vi "test.vi"() -> ()   [LabVIEW 2010, in "GenericAnalogOut.lvclass"]
uses:
  GenericAnalogOut.lvclass
  common/classes/ErrorController/ErrorController/ErrorController.lvclass
  common/classes/ErrorController/ErrorController/class_data.vi
  common/classes/GenericComponent/GenericComponent/GenericComponent.lvclass
panel:
  out "error loaded?":bool
  in  "create button":bool
  in  "set button":bool
  in  "output voltage":dbl[unit]
  in  "stop button":bool
  # "Test panel for AnalogOut components"
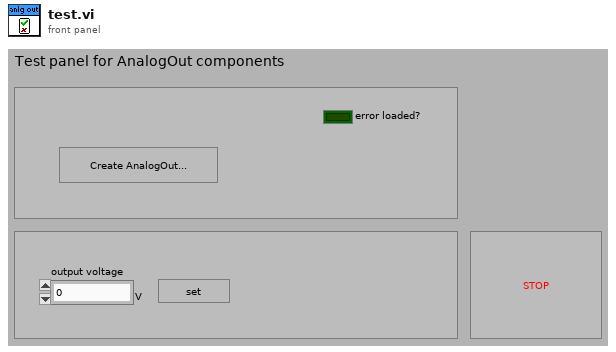
[diagram p1: front panel]
types:
  T1 = typedef "XComponentSpecification.xctl/data.ctl" = cluster{"class path":string, "configuration":string, "label":string, "settings name":string}
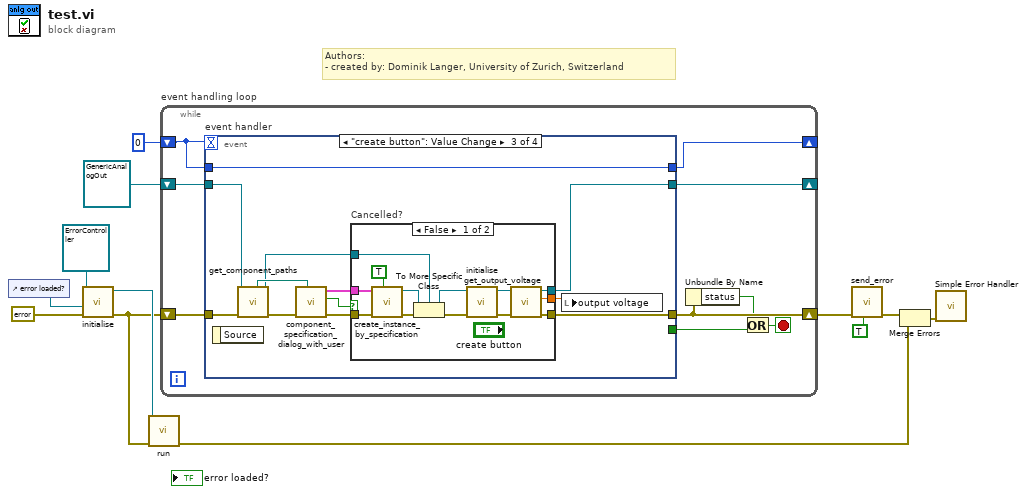
[diagram p0: block diagram]
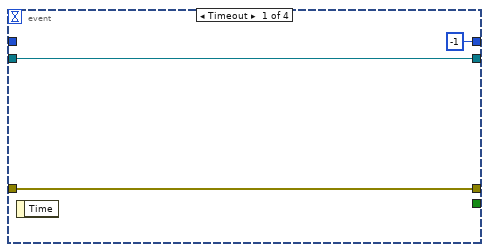
[diagram p2: hidden frame]
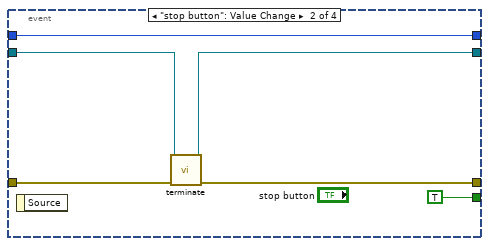
[diagram p3: hidden frame]
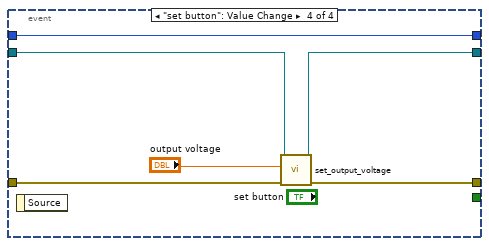
[diagram p5: hidden frame]
diagram:
  # "Authors: \n- created by: Dominik Langer, University of Zurich, Switzerland"
  n1 = control-ref of="error loaded?"() -> (w9:refnum<vi>)
  n2 = call-dynamic "initialise.vi"("error in (no error)"=errorcluster {"status"=FALSE, "code"=0, "source"=""} ("error out"), "error boolean"=w9, "ErrorController in"=refnum<class "ErrorController.lvclass"> refnum ("ErrorController.lvclass")) -> ("error out"=w2:errorcluster, "ErrorController out"=w8:refnum<class "ErrorController.lvclass">)  [unwired: 7 in]
  n3 = call "run.vi"("error in (no error)"=w2, "ErrorController in"=w8) -> ("error out"=w3:errorcluster)  [unwired: 8 in, 1 out]
  n4 = while "event handling loop" {
    shift-right: [w16] -> w7
    shift-left: w2 -> [w21]
    shift-right: [w19] -> _
    shift-left: 0 -> [w20]
    shift-right: [w17] -> _
    shift-left: refnum<class "GenericAnalogOut.lvclass"> refnum ("GenericAnalogOut.lvclass") -> [w18]
    stop <- w13 stop-if-true
    n5 = event "event handler" shown="[2] \"create button\": Value Change" {
      selector: _ -> [_ _ _ _]
      dyn-events: _ -> [_ _ _ _]
      timeout: w20 -> [_ _ _ _]
      tunnel: w21 -> [w23 w26 w36 w62]
      tunnel: [w23 w25 w40 w61] -> w16
      tunnel: [-1 w30 w42 w63] -> w19
      tunnel: w20 -> [_ w30 w42 w63]
      tunnel: w18 -> [w22 w28 w34 w60]
      tunnel: [w22 w27 w39 w59] -> w17
      tunnel: [_ TRUE _ _] -> w14
      event Timeout {
        n6 = event-data() -> ()  [unwired: 2 out]
      }
      event "stop button": Value Change {
        n7 = event-data() -> ()  [unwired: 2 out]
        n8 = call-dynamic "terminate.vi"("error in (no error)"=w26, "GenericPlugin in"=w28) -> ("error out"=w25:errorcluster, "GenericPlugin out"=w27:refnum<class "GenericAnalogOut.lvclass">)  [unwired: 8 out]
      }
      event "create button": Value Change {
        n9 = event-data() -> ()  [unwired: 2 out]
        n10 = call-dynamic "get_component_paths.vi"("error in (no error)"=w36, "GenericComponent in"=w34) -> ("error out"=w38:errorcluster, "GenericComponent out"=w33:refnum<class "GenericAnalogOut.lvclass">, "component type directory"=w37:path)  [unwired: 4 in, 3 out]
        n11 = call "component_specification_dialog_with_user.vi"("start path"=w37, "error in (no error)"=w38) -> ("error out"=w35:errorcluster, "cancelled?"=w32:bool, "component specification out"=w31:T1)  [unwired: 7 in]
        n12 = case "Cancelled?" shown="False" w32 {
          tunnel: [w53 _] -> w41
          tunnel: [w52 w56] -> w40
          tunnel: [w51 w57] -> w39
          tunnel: w35 -> [w50 w56]
          tunnel: w33 -> [w47 w57]
          tunnel: w31 -> [w49 _]
          frame False {
            n13 = call "create_instance_by_specification.vi"("call constructor?"=TRUE, "error in (no error)"=w50, "component specification"=w49) -> ("error out"=w48:errorcluster, "GenericPlugin out"=w46:refnum<class "GenericComponent.lvclass">)  [unwired: 6 in, 1 out]
            n14 = To More Specific Class(target class=w47, reference=w46, error in=w48) -> (specific class reference=w44:refnum<class "GenericAnalogOut.lvclass">, error out=w43:errorcluster)
            n15 = call-dynamic "initialise.vi"("error in (no error)"=w43, "GenericPlugin in"=w44) -> ("error out"=w55:errorcluster, "GenericPlugin out"=w54:refnum<class "GenericAnalogOut.lvclass">)  [unwired: 8 out]
            n16 = call-dynamic "get_output_voltage.vi"("error in (no error)"=w55, "GenericAnalogOut in"=w54) -> ("error out"=w52:errorcluster, "current voltage"=w53:dbl[unit], "GenericAnalogOut out"=w51:refnum<class "GenericAnalogOut.lvclass">)  [unwired: 7 in]
          }
          frame True {
          }
        }
        n17 = local write "output voltage"(w41) -> ()
      }
      event "set button": Value Change {
        n18 = event-data() -> ()  [unwired: 2 out]
        n19 = call-dynamic "set_output_voltage.vi"("error in (no error)"=w62, "output value"="output voltage", "GenericAnalogOut in"=w60) -> ("error out"=w61:errorcluster, "GenericAnalogOut out"=w59:refnum<class "GenericAnalogOut.lvclass">)  [unwired: 7 in]
      }
    }
    n20 = Unbundle By Name(w16) -> ("status"=w15:bool)
    n21 = Or(x=w15, y=w14) -> (x .or. y?=w13:bool)
  }
  n22 = call "send_error.vi"("last error? (F)"=TRUE, "error in (no error)"=w7) -> ("error out"=w6:errorcluster)  [unwired: 9 in]
  n23 = Merge Errors(w6, w3) -> (w4:errorcluster)
  n24 = call <vilib>:"Simple Error Handler.vi"("error in (no error)"=w4) -> ()  [unwired: 1 in, 8 out]
